vi "saveLogToFile.vi"(8 "error in (no error)":errorcluster, 11 "Log in":refnum<class "Log.lvclass">) -> (0 "error out":errorcluster, 3 "Log out":refnum<class "Log.lvclass">)   [LabVIEW 2011, in "Tools.lvlib" / "xml.lvlib" / "Log.lvclass"]
uses:
  Log.lvclass
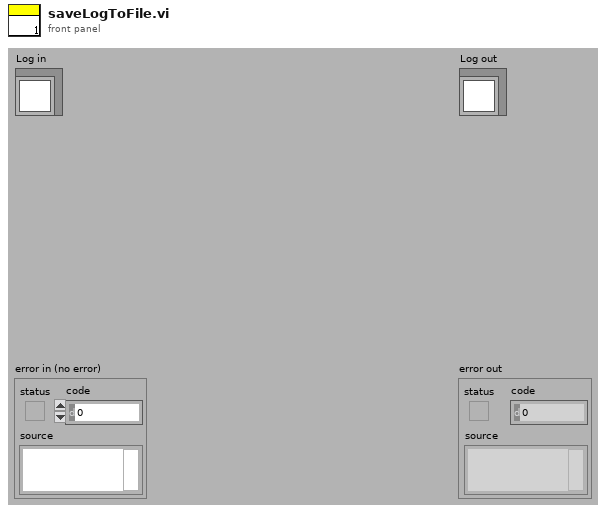
[diagram p1: front panel]
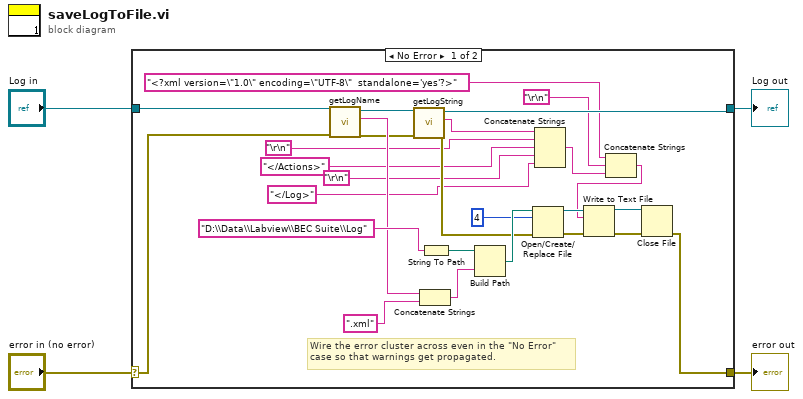
[diagram p0: block diagram]
diagram:
  n1 = case shown="No Error" "error in (no error)" {
    selector: "error in (no error)" -> [w26 w33]
    tunnel: [w19 w33] -> w3
    tunnel: [w22 w32] -> w1
    tunnel: "Log in" -> [w25 w32]
    frame No Error {
      # "Wire the error cluster across even in the \"No Error\"\ncase so that warnings get propagated."
      n2 = call-dynamic "getLogName.vi"("error in (no error)"=w26, "Log.lvclass in"=w25) -> ("error out"=w23:errorcluster, "logName"=w27:string, "Log.lvclass out"=w24:refnum<class "Log.lvclass">)  [unwired: 7 in]
      n3 = call-dynamic "getLogString.vi"("error in (no error)"=w23, "Log.lvclass in"=w24) -> ("error out"=w15:errorcluster, "logString"=w13:string, "Log.lvclass out"=w22:refnum<class "Log.lvclass">)  [unwired: 7 in]
      n4 = Concatenate Strings(w27, ".xml") -> (w29:string)
      n5 = String To Path(string="D:\\Data\\Labview\\BEC Suite\\Log") -> (path=w31:path)
      n6 = Build Path(base path=w31, name or relative path=w29) -> (appended path=w16:path)
      n7 = Open/Create/Replace File(file path (use dialog)=w16, error in=w15, operation (0:open)=4) -> (refnum out=w18:refnum<file>, error out=w17:errorcluster)  [unwired: 3 in, 1 out]
      n8 = Concatenate Strings(w13, "\r\n", "</Actions>", "\r\n", "</Log>") -> (w9:string)
      n9 = Concatenate Strings("<?xml version=\"1.0\" encoding=\"UTF-8\"  standalone='yes'?>", "\r\n", w9) -> (w6:string)
      n10 = Write to Text File(file (use dialog)=w18, text=w6, error in=w17) -> (refnum out=w20:refnum<file>, error out=w21:errorcluster)  [unwired: 1 in, 1 out]
      n11 = Close File(refnum=w20, error in=w21) -> (error out=w19:errorcluster)  [unwired: 1 out]
    }
    frame Error {
    }
  }
  "error out" <- w3
  "Log out" <- w1
